vi "VI Snippet Import.vi"(6 "App Refnum (New VI only)":refnum<vi>, 7 "Copy to (\"VI\")":enum8{"VI", "Clipboard"}(ring), 8 "error in (no error)":errorcluster, 9 "Drop Position (0, 0)":cluster{"Left":i32, "Top":i32}, 10 "VI Refnum in (NaN=New VI)":refnum<vi>, 11 "VI Snippet Path (*.png)":path) -> (0 "error out":errorcluster, 1 "New VI?":bool, 2 "Image Data out":T1, 3 "VI Refnum out":refnum<vi>)   [LabVIEW 2019, in "VI Snippet.lvlib"]
doc: "Import a VI Snippet from the <b>VI Snippet Path (*.png)</b>. Set <b>Copy to</b> as either <b>\"VI\"</b> or <b>\"Clipboard\"</b> to copy the VI Snippet content to a existing/new VI (<b>VI Refnum/NaN</b>) or copy the content to the clipboard. By default, this copies the VI Snippet to a new VI. Specify the <b>Drop Position</b> when placing content into an existing VI. The <b>Drop Position</b> has no effect for new VIs. <b>Copy to</b> <b>\"Clipboard\"</b> does not return a <b>VI Refnum out</b>. \n\n<b>Errors:</b>\n<b>1430: \"Empty path\"</b> is raised if the <b>VI Snippet Path (*.png)</b> is empty or not a path.\n\nCreated by: Ryan Pacini"
uses:
  VI Snippet.lvlib
  <vilib>/picture/picture.llb/imagedata.ctl
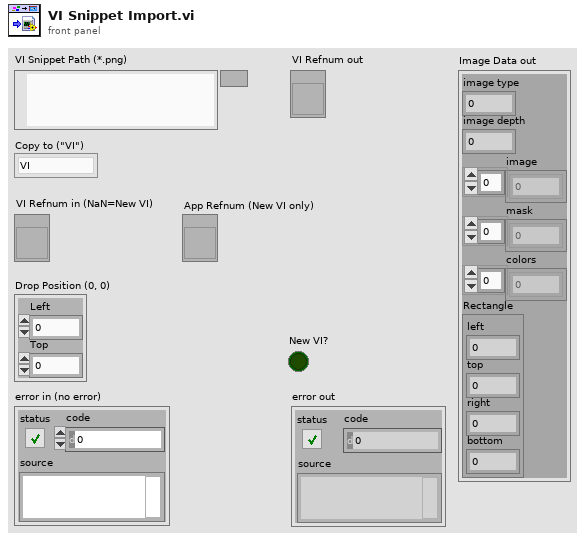
[diagram p1: front panel]
types:
  T1 = typedef "imagedata.ctl" = cluster{"image type":i32, "image depth":i32, "image":u8[], "mask":u8[], "colors":u32[], "Rectangle":cluster{"left":i16, "top":i16, "right":i16, "bottom":i16}}
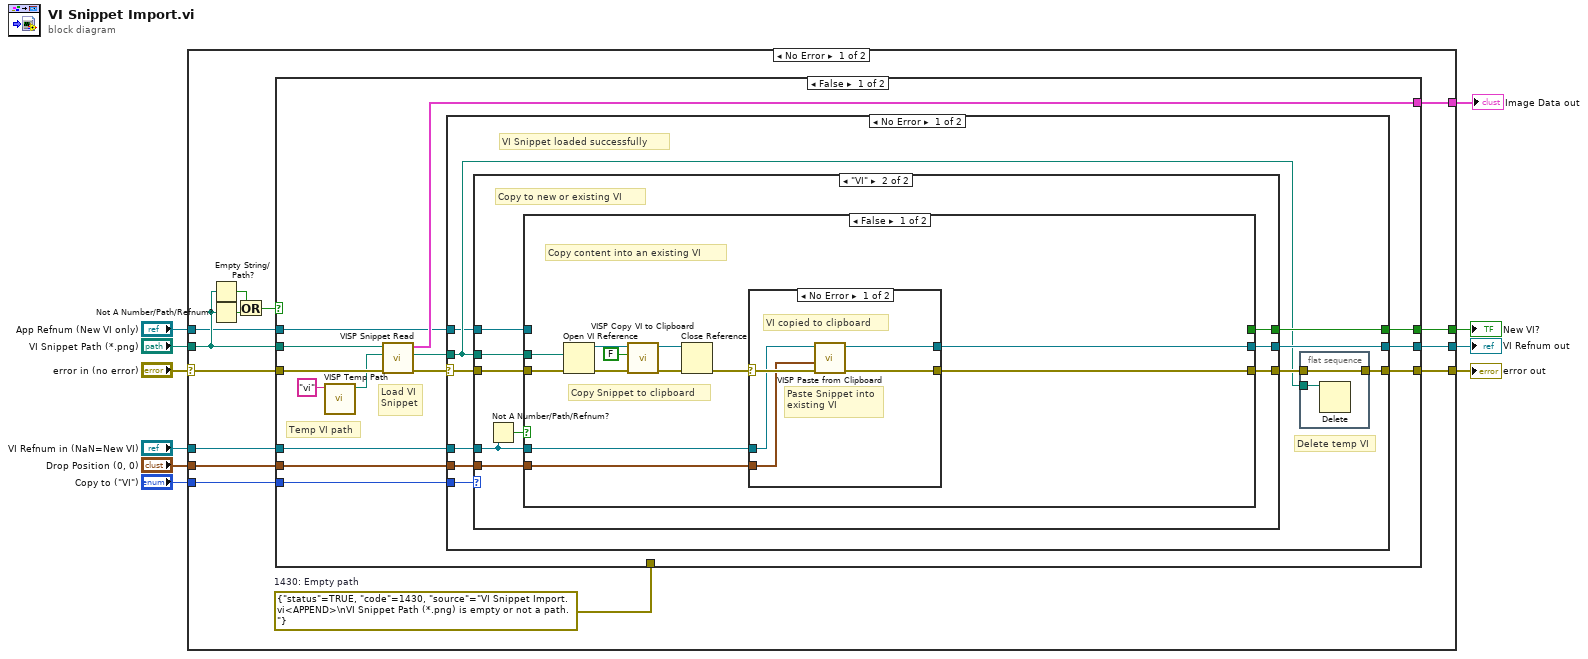
[diagram p0: block diagram]
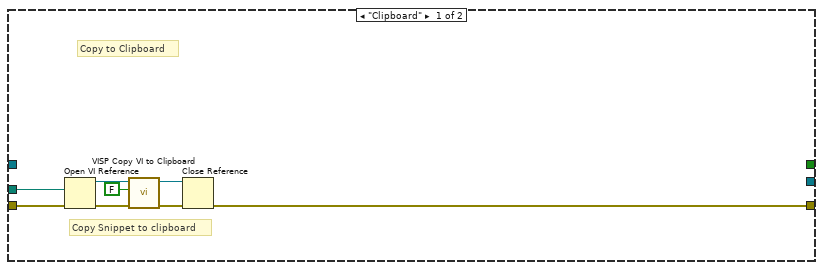
[diagram p2: hidden frame]
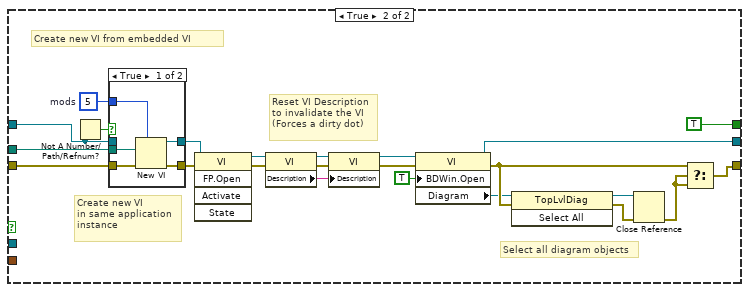
[diagram p4: hidden frame]
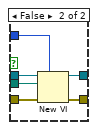
[diagram p5: hidden frame]
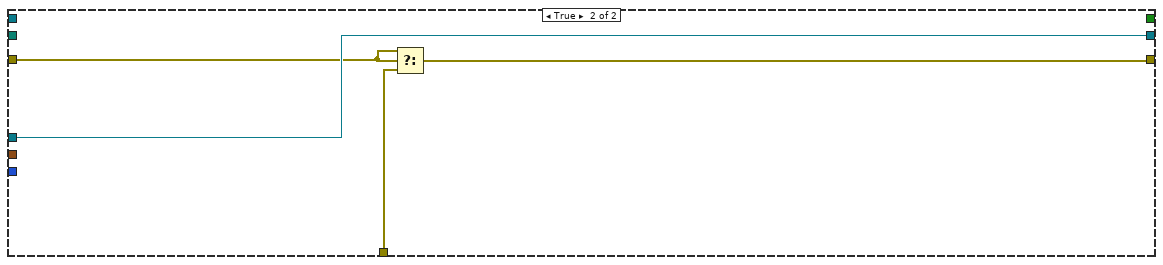
[diagram p7: hidden frame]
diagram:
  n1 = case shown="No Error" "error in (no error)" {
    selector: "error in (no error)" -> [w19 w128]
    tunnel: "VI Snippet Path (*.png)" -> [w15 _]
    tunnel: "VI Refnum in (NaN=New VI)" -> [w24 w127]
    tunnel: "Drop Position (0, 0)" -> [w23 _]
    tunnel: [w22 w128] -> w7
    tunnel: [w21 w127] -> w5
    tunnel: [w20 _] -> w4
    tunnel: [w18 _] -> w3
    tunnel: "Copy to (\"VI\")" -> [w12 _]
    tunnel: "App Refnum (New VI only)" -> [w11 _]
    frame No Error {
      w13 = errorcluster {"status"=TRUE, "code"=1430, "source"="VI Snippet Import.vi<APPEND>\nVI Snippet Path (*.png) is empty or not a path."}  # 1430: Empty path
      n2 = Empty String/Path?(string/path=w15) -> (empty?=w17:bool)
      n3 = Not A Number/Path/Refnum?(number/path/refnum=w15) -> (NaN/Path/Refnum?=w16:bool)
      n4 = Or(x=w17, y=w16) -> (x .or. y?=w14:bool)
      n5 = case shown="False" w14 {
        tunnel: w24 -> [w38 w126]
        tunnel: w23 -> [w37 _]
        tunnel: [w36 w125] -> w22
        tunnel: [w35 w126] -> w21
        tunnel: [w34 _] -> w20
        tunnel: w19 -> [w33 w124]
        tunnel: w15 -> [w30 _]
        tunnel: [w28 _] -> w18
        tunnel: w13 -> [_ w123]
        tunnel: w12 -> [w26 _]
        tunnel: w11 -> [w25 _]
        frame False {
          # "Temp VI path"
          # "Load VI\nSnippet"
          n6 = call "VISP Temp Path.vi"("Extension (\"vi\")"="vi" ("Temporary File Extension (tmp)")) -> ("Path (*.png)"=w27:path)  [unwired: 10 in]
          n7 = call "VISP Snippet Read.vi"("error in (no error)"=w33, "VI Path (*.vi)"=w27, "VI Snippet Path (*.png)"=w30) -> ("error out"=w32:errorcluster, "dup VI Path"=w29:path, "Image Data out"=w28:T1)  [unwired: 6 in]
          n8 = case shown="No Error" w32 {
            selector: w32 -> [w45 w121]
            tunnel: w38 -> [w44 w122]
            tunnel: w37 -> [w48 _]
            tunnel: [w42 w121] -> w36
            tunnel: [w47 w122] -> w35
            tunnel: [w46 _] -> w34
            tunnel: w29 -> [w41 _]
            tunnel: w26 -> [w40 _]
            tunnel: w25 -> [w39 _]
            frame No Error {
              # "Delete temp VI"
              # "VI Snippet loaded successfully"
              n9 = case shown="\"VI\"" w40 {
                tunnel: w48 -> [_ w65]
                tunnel: [_ w64] -> w47
                tunnel: [_ w63] -> w46
                tunnel: w45 -> [w51 w62]
                tunnel: w44 -> [_ w61]
                tunnel: [w49 w59] -> w43
                tunnel: w41 -> [w50 w58]
                tunnel: w39 -> [_ w57]
                frame "Clipboard" {
                  # "Copy to Clipboard"
                  # "Copy Snippet to clipboard"
                  n10 = Open VI Reference(vi path=w50, error in (no error)=w51) -> (vi reference=w54:refnum<vi>, error out=w55:errorcluster)  [unwired: 4 in]
                  n11 = call "VISP Copy VI to Clipboard.vi"("error in (no error)"=w55, "Selected GObjects Only? (F)"=FALSE, "VI Refnum in"=w54) -> ("error out"=w56:errorcluster, "dup VI Refnum"=w53:refnum<vi>)  [unwired: 7 in]
                  n12 = Close Reference(reference=w53, error in (no error)=w56) -> (error out=w49:errorcluster)
                }
                frame "VI" {
                  # "Copy to new or existing VI"
                  n13 = Not A Number/Path/Refnum?(number/path/refnum=w61) -> (NaN/Path/Refnum?=w60:bool)
                  n14 = case shown="False" w60 {
                    tunnel: w61 -> [w77 _]
                    tunnel: w65 -> [w76 _]
                    tunnel: [w75 w98] -> w59
                    tunnel: [w74 w91] -> w64
                    tunnel: [_ TRUE ("New VI?")] -> w63
                    tunnel: w62 -> [w73 w107]
                    tunnel: w58 -> [w67 w102]
                    tunnel: w57 -> [_ w95]
                    frame False {
                      # "Copy content into an existing VI"
                      # "Copy Snippet to clipboard"
                      n15 = Open VI Reference(vi path=w67, error in (no error)=w73) -> (vi reference=w70:refnum<vi>, error out=w71:errorcluster)  [unwired: 4 in]
                      n16 = call "VISP Copy VI to Clipboard.vi"("error in (no error)"=w71, "Selected GObjects Only? (F)"=FALSE, "VI Refnum in"=w70) -> ("error out"=w72:errorcluster, "dup VI Refnum"=w69:refnum<vi>)  [unwired: 7 in]
                      n17 = Close Reference(reference=w69, error in (no error)=w72) -> (error out=w66:errorcluster)
                      n18 = case shown="No Error" w66 {
                        selector: w66 -> [w82 w84]
                        tunnel: w77 -> [w78 w83]
                        tunnel: w76 -> [w81 _]
                        tunnel: [w80 w84] -> w75
                        tunnel: [w79 w83] -> w74
                        frame No Error {
                          # "VI copied to clipboard"
                          # "Paste Snippet into\nexisting VI"
                          n19 = call "VISP Paste from Clipboard.vi"("error in (no error)"=w82, "Drop Position (0, 0)"=w81, "VI Refnum in"=w78) -> ("error out"=w80:errorcluster, "VI Refnum out"=w79:refnum<vi>)  [unwired: 7 in]
                        }
                        frame Error {
                          # "Failed to copy \nVI Snippet to clipboard"
                        }
                      }
                    }
                    frame True {
                      w93 = u32 5  # mods
                      # "Reset VI Description\nto invalidate the VI\n(Forces a dirty dot)"
                      # "Select all diagram objects"
                      # "Create new VI\nin same application\ninstance"
                      # "Create new VI from embedded VI"
                      n20 = Not A Number/Path/Refnum?(number/path/refnum=w95) -> (NaN/Path/Refnum?=w94:bool)
                      n21 = case shown="True" w94 {
                        tunnel: w107 -> [w112 w118]
                        tunnel: [w111 w117] -> w106
                        tunnel: [w110 w116] -> w92
                        tunnel: w102 -> [w109 w115]
                        tunnel: w95 -> [_ w114]
                        tunnel: w93 -> [w108 w113]
                        frame True {
                          n22 = New VI(7:w108, 8:w112, 10:w109) -> (0:w111:errorcluster, 3:w110:refnum<vi>)  [unwired: 4 in]
                        }
                        frame False {
                          n23 = New VI(7:w113, 8:w118, 10:w115, 11:w114) -> (0:w117:errorcluster, 3:w116:refnum<vi>)  [unwired: 3 in]
                        }
                      }
                      n24 = invoke class="VI" method="FP.Open"(reference=w92, error in=w106) -> (reference out=w105:refnum<vi>, error out=w90:errorcluster)  [unwired: 3 in, 3 out]
                      n25 = property class="VI"(reference=w105, error in=w90) -> (reference out=w89:refnum<vi>, error out=w88:errorcluster, "Description"=w85:string)
                      n26 = property class="VI"(reference=w89, error in=w88, "Description"=w85) -> (reference out=w86:refnum<vi>, error out=w87:errorcluster)
                      n27 = property class="VI"(reference=w86, error in=w87, "BDWin.Open"=TRUE ("Block Diagram Window:Open")) -> (reference out=w91:refnum<vi>, error out=w97:errorcluster, "Diagram"=w96:refnum<vi>)
                      n28 = invoke class="TopLvlDiag" method="Select All"(reference=w96, error in=w97) -> (reference out=w101:refnum<vi>, error out=w100:errorcluster)  [unwired: 1 in, 1 out]
                      n29 = Close Reference(reference=w101, error in (no error)=w100) -> (error out=w99:errorcluster)
                      n30 = Select(t=w97, s=w99, f=w99) -> (s? t:f=w98:errorcluster)
                    }
                  }
                }
              }
              n31 = flat-sequence {
                tunnel: w41 -> [w120]
                tunnel: [w119] -> w42
                tunnel: w43 -> [w119]
                frame #0 {
                  n32 = Delete(path (use dialog)=w120) -> ()  [unwired: 4 in, 3 out]
                }
              }
            }
            frame Error {
              # "Failed to load VI Snippet"
            }
          }
        }
        frame True {
          n33 = Select(t=w124, s=w124, f=w123) -> (s? t:f=w125:errorcluster)
        }
      }
    }
    frame Error {
    }
  }
  "error out" <- w7
  "VI Refnum out" <- w5
  "New VI?" <- w4
  "Image Data out" <- w3
